vi "Waveform Graph Data Types.vi"() -> ()   [LabVIEW 2018]
doc: "Illustrates the various single plot and multi plot data types that the waveform graph accepts. Use the waveform graph to display data that is uniformly distributed along the X-axis. This is particularly useful when displaying data that was sampled at a uniform rate."
panel:
  in  "Tab Control":enum32{"Default Time base", "Custom Time bases"}(tab)
  out "Single Plot":dbl[](graph)
  out "Multiple Plots":dbl[][](graph)
  out "Single Plot (custom time base)":cluster{"xo":i32, "dx":i32, dbl[]}(graph)
  out "Multiple Plots (custom time base)":cluster{"xo":i32, "dx":i32, dbl[][]}(graph)
  # "Overview: Demonstrates various waveform graph data types.\nInstructions:\n1. Run the VI.\n2. Switch between the tabs to observe the appearance of the various waveform graphs."
  # "Waveform graphs that use data indices for the X-axis are array data types on the block diagram."
  # "These graphs use the index values of the displayed data for X-axis values.  So the first value in the data array has an X-axis value of '0', the second value in the data array has an X-axis value of '1', etc. This is the default mode of operation and data display for the Waveform Graph."
  # "Waveform graphs that use custom time base values for the X-axis are cluster data types on the block diagram."
  # "These graphs use a custom time base for the X-Axis, as defined by the clusters on the diagram. Specifically, these graphs have been given an initial X-Axis value of '10', and a delta between successive X-Axis values of '2'."
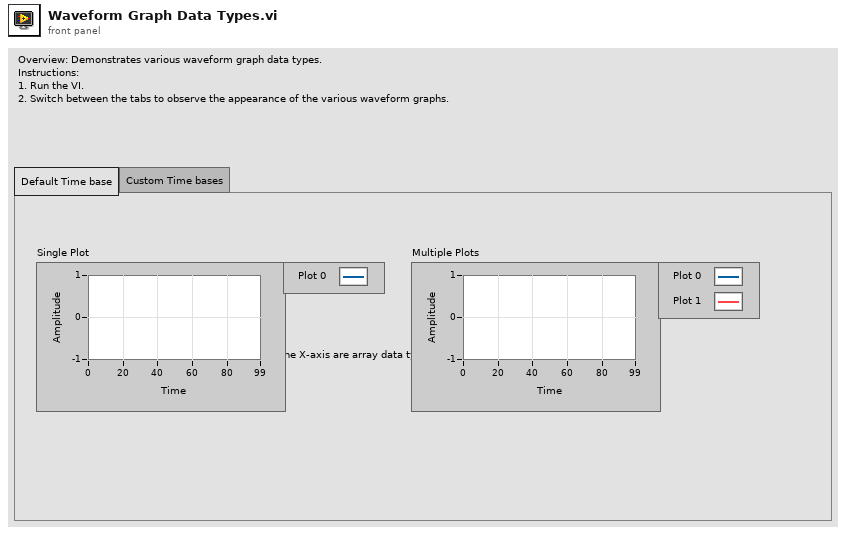
[diagram p1: front panel]
types:
  T1 = cluster{"Initial X-Axis Value":i32, "Delta X":i32, dbl[]}
  T2 = cluster{"Initial X-Axis Value":i32, "Delta X":i32, dbl[][]}
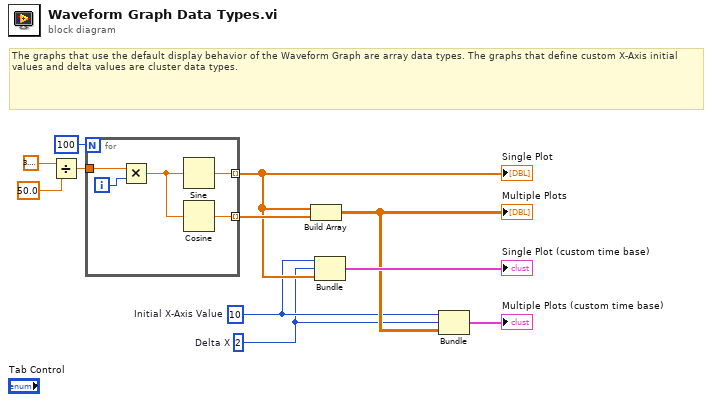
[diagram p0: block diagram]
diagram:
  w1 = 2  # Delta X
  w2 = 10  # Initial X-Axis Value
  # "The graphs that use the default display behavior of the Waveform Graph are array data types. The graphs that define custom X-Axis initial values and delta values are cluster data types."
  n1 = Divide(x=3.141592653589793, y=50.0) -> (x/y=w9:dbl)
  n2 = for {
    N: 100 -> [_]
    tunnel: w9 -> [w16]
    tunnel: [w14] -> w6 mode=indexing
    tunnel: [w13] -> w8 mode=indexing
    i -> [w12]
    n3 = Multiply(x=w16, y=w12) -> (x*y=w15:dbl)
    n4 = Sine(x=w15) -> (sin(x)=w14:dbl)
    n5 = Cosine(x=w15) -> (cos(x)=w13:dbl)
  }
  "Single Plot" <- w6
  n6 = Build Array(w6, w8) -> (w4:dbl[][])
  "Multiple Plots" <- w4
  n7 = Bundle("Initial X-Axis Value"=w2, "Delta X"=w1, w6) -> (→"Single Plot (custom time base)":T1)  [unwired: 1 in]
  n8 = Bundle("Initial X-Axis Value"=w2, "Delta X"=w1, w4) -> (→"Multiple Plots (custom time base)":T2)  [unwired: 1 in]
